vi "Set Setpoint.vi"(7 "Select Channel":i32=1 min=1 max=4 step=1, 8 "error in (no error)":errorcluster, 10 "Setpoint":dbl, 11 "Temp Control in":refnum<class "Temp Control.lvclass">) -> (0 "error out":errorcluster, 3 "Temp Control out":refnum<class "Temp Control.lvclass">)   [LabVIEW 2022 SP3, in "Temp Control.lvclass"]
uses:
  Temp Control.lvclass
  Temp Control.lvclass/Temp Control.ctl
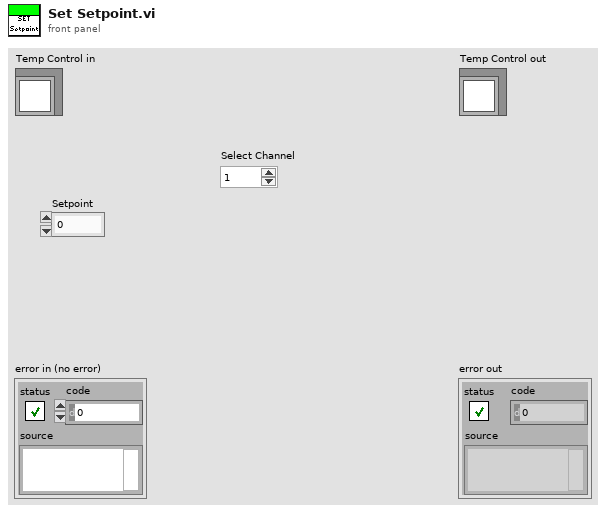
[diagram p1: front panel]
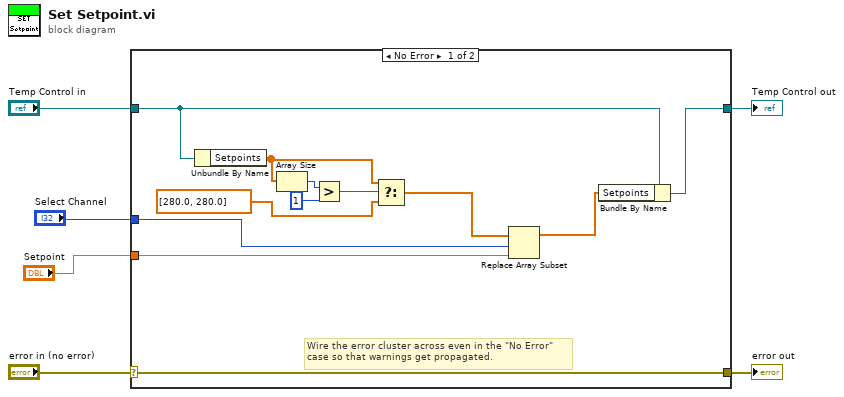
[diagram p0: block diagram]
diagram:
  n1 = case shown="No Error" "error in (no error)" {
    selector: "error in (no error)" -> [w18 w20]
    tunnel: [w18 w20] -> w5
    tunnel: [w17 w19] -> w3
    tunnel: "Temp Control in" -> [w16 w19]
    tunnel: "Setpoint" -> [w15 _]
    tunnel: "Select Channel" -> [w14 _]
    frame No Error {
      # "Wire the error cluster across even in the \"No Error\"\ncase so that warnings get propagated."
      n2 = Unbundle By Name(w16) -> ("Setpoints"=w8:dbl[])
      n3 = Array Size(array=w8) -> (size(s)=w12:i32)
      n4 = Greater?(x=w12, y=1) -> (0:w10:bool)
      n5 = Select(t=w8, s=w10, f=dbl[] [280.0, 280.0] ("Setpoints")) -> (s? t:f=w7:dbl[])
      n6 = Replace Array Subset(array=w7, new element=w15, index=w14) -> (w13:dbl[])
      n7 = Bundle By Name(cluster=w16, "Setpoints"=w13) -> (w17:refnum<class "Temp Control.lvclass">)
    }
    frame Error {
    }
  }
  "error out" <- w5
  "Temp Control out" <- w3
